vi "Output Select and EnableMod.vi"(8 "error in (no error)":errorcluster, 10 "streaming output.threshold":u32, 11 "Refnum in":refnum<k20>) -> (0 "error out":errorcluster, 3 "Refnum out":refnum<k20>)   [LabVIEW 2017]
uses:
  <vilib>/Utility/error.llb/Error Cluster From Error Code.vi
  <vilib>/rvi/errors/niLvFpgaAdjustHostInterfaceError.vi
  <vilib>/rvi/interface/nirviReadWriteControl/nirviReadWriteControl.xnode
  NiFpgaLv.dll
  <vilib>/rvi/interface/Simulation/niFpgaSimulationCallBeginRW.vi
panel:
  out "streaming output.dma fullness":u32
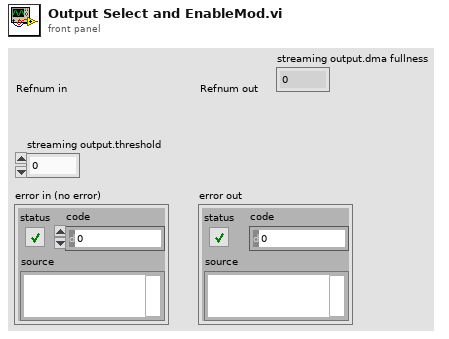
[diagram p1: front panel]
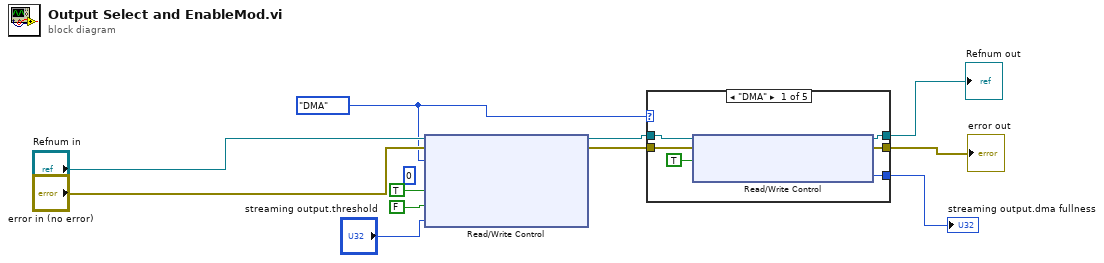
[diagram p0: block diagram]
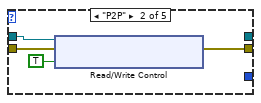
[diagram p2: hidden frame]
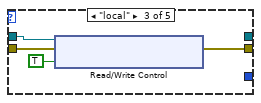
[diagram p3: hidden frame]
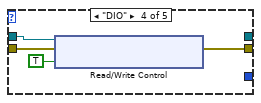
[diagram p4: hidden frame]
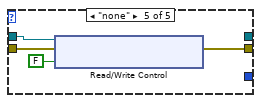
[diagram p5: hidden frame]
diagram:
  (unwired) u32 0 ("streaming output.burst size")
  w1 = enum16{"none", "DMA", "local", "P2P", "DIO"}."DMA" ("stream select")
  n1 = xnode "Read/Write Control"("FPGA VI Reference In"="Refnum in", "error in"="error in (no error)", "streaming output.select"=w1, "streaming output.reset"=TRUE, "streaming output.reset"=FALSE, "streaming output.threshold"="streaming output.threshold") -> ("FPGA VI Reference Out"=w6:refnum<k20>, "error out"=w5:errorcluster)  [unwired: 1 in]
  n2 = case shown="\"DMA\"" w1 {
    tunnel: w5 -> [w16 w20 w24 w28 w32]
    tunnel: w6 -> [w17 w21 w25 w29 w33]
    tunnel: [w14 w18 w22 w26 w30] -> w9
    tunnel: [w13 _ _ _ _] -> w2
    tunnel: [w12 _ _ _ _] -> w8
    frame "DMA" {
      n3 = xnode "Read/Write Control"("FPGA VI Reference In"=w17, "error in"=w16, "streaming output.enable"=TRUE) -> ("FPGA VI Reference Out"=w12:refnum<k20>, "error out"=w14:errorcluster, "streaming output.dma fullness"=w13:u32)
    }
    frame "P2P" {
      n4 = xnode "Read/Write Control"("FPGA VI Reference In"=w21, "error in"=w20, "streaming output.enable"=TRUE) -> ("error out"=w18:errorcluster)  [unwired: 1 out]
    }
    frame "local" {
      n5 = xnode "Read/Write Control"("FPGA VI Reference In"=w25, "error in"=w24, "streaming output.enable"=TRUE) -> ("error out"=w22:errorcluster)  [unwired: 1 out]
    }
    frame "DIO" {
      n6 = xnode "Read/Write Control"("FPGA VI Reference In"=w29, "error in"=w28, "streaming output.enable"=TRUE) -> ("error out"=w26:errorcluster)  [unwired: 1 out]
    }
    frame "none" {
      n7 = xnode "Read/Write Control"("FPGA VI Reference In"=w33, "error in"=w32, "streaming output.enable"=FALSE) -> ("error out"=w30:errorcluster)  [unwired: 1 out]
    }
  }
  "error out" <- w9
  "Refnum out" <- w8
  "streaming output.dma fullness" <- w2
